vi "List Managers.vi"(10 "Include Cache? (F)":bool, 11 "SMOConfigManagerCollection in":refnum<class "ConfigManagerCollection.lvclass">) -> (2 "List":refnum<class "ConfigManager.lvclass">[](array[class]), 3 "SMOConfigManagerCollection out":refnum<class "ConfigManagerCollection.lvclass">)   [LabVIEW 2013, in "CfgManager.lvlib" / "ConfigManagerCollection.lvclass"]
uses:
  ConfigManagerCollection.lvclass
  Manager/ConfigManager.lvclass
  ConfigManagerCollection.lvclass/ConfigManagerCollection.ctl
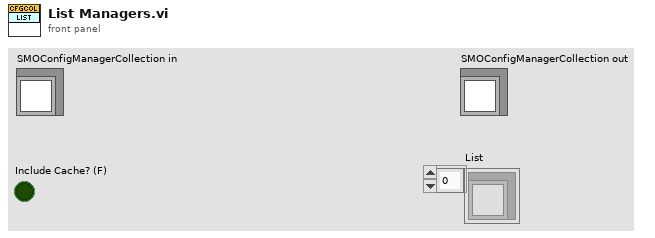
[diagram p1: front panel]
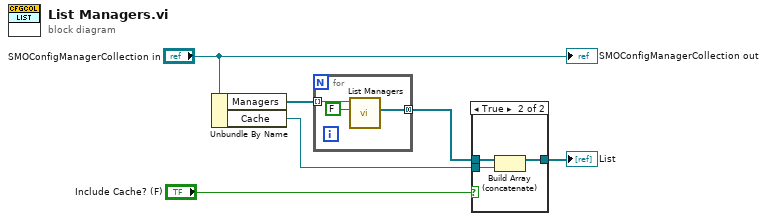
[diagram p0: block diagram]
diagram:
  n1 = Unbundle By Name("SMOConfigManagerCollection in") -> ("Managers"=w5:refnum<class "ConfigManager.lvclass">[], "Cache"=w4:refnum<class "ConfigManager.Cache.lvclass">)
  n2 = for {
    tunnel: w5 -> [w9] mode=indexing
    tunnel: [w8] -> w2 mode=concatenating
    n3 = call-dynamic "List Managers.vi"("Include Cache? (F)"=FALSE, "SMOConfigManager in"=w9) -> ("List"=w8:refnum<class "ConfigManager.lvclass">[])  [unwired: 8 in, 1 out]
  }
  n4 = case shown="True" "Include Cache? (F)" {
    tunnel: w4 -> [_ w13]
    tunnel: [w10 w12] -> w3
    tunnel: w2 -> [w10 w11]
    frame False {
    }
    frame True {
      n5 = Build Array (concatenate)(w11, w13) -> (w12:refnum<class "ConfigManager.lvclass">[])
    }
  }
  "List" <- w3
  "SMOConfigManagerCollection out" <- "SMOConfigManagerCollection in"
